vi "Emballage FLATPROP.vi"(2 "error in (no error)":errorcluster caption="entrée d'erreur (pas d'erreur)") -> (0 "error out":errorcluster={"status"=TRUE, "code"=-1, "source"="Fichier des listes de produit vide"} caption="sortie d'erreur")   [LabVIEW 2020]
uses:
  Modules/FS/60_FS_Controles/60_FS_SetGet.ctl
  Labview emballage/enum_ON_OFF_Lecteur.ctl
  41349739-ea89-4dfa-8987-3cac980ec602.vi
  <vilib>/Array/Sort 2D Array - Pop Stack.vi
  <vilib>/Array/Sort 2D Array - Push Stack.vi
  Instance          16 21Saved   Emballage V08 .vi
panel:
  out "Nbr p. dernier carton":i16
  out "NumSem":dbl
  out "Version":string caption="String"
  in  "Certificat":bool
  out "Continuer l'emballage":bool
  out "arreterSerie":bool
  out "pièces EC emballées":string
  out "offset sur code \nbar début index":i32
  out "largeur index":i32
  out "Série en cours?":bool
  out "n° lot à scanner":string
  out "recommencer la cmde EC":bool
  out "#valve déjà emballée":i32
  out "Tableau lots OUT":string[][](array[string])
  out "index commande en cours":i32
  out "Etat":T1(ring)
  out "ID Employe":string
  out "Commande interne":bool
  in  "Imprimer n° cmde":bool
  out "Commande":string
  in  "quitter":bool
  in  "historique":bool
  in  "EC emballage":bool
  in  "carton":bool
  out "Article":string
  out "Nom":string
  out "Nombre de pièce":i16
  out "Numéro carton":i16
  out "Numéro scanné":string
  # "Emballage BDD"
  # "Init"
  # "VerificationSerie"
  # "PieceScannee"
  # "VerificationSerie"
  # "Version"
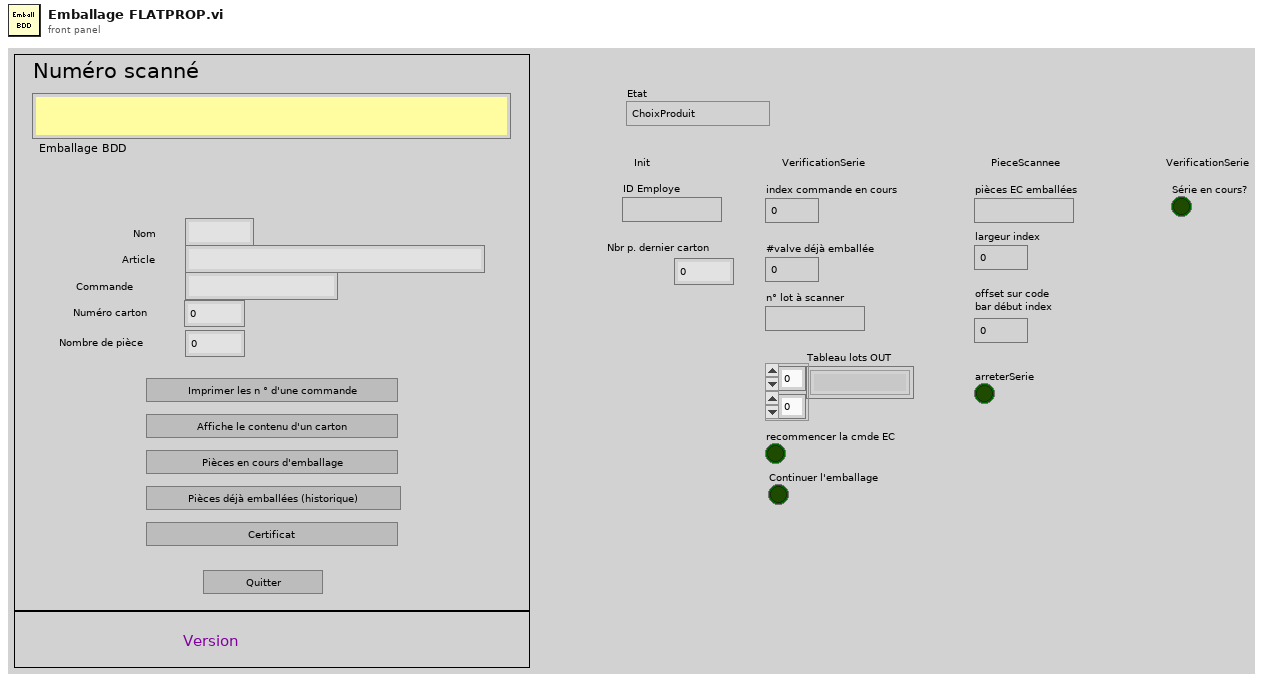
[diagram p1: front panel]
types:
  T1 = enum16{"ChoixProduit", "Init", "VerificationSerie", "LecteurON", "PieceScannee", "LecteurOFF", "SaveData"}
  T2 = typedef "60_FS_SetGet.ctl" = enum16{"set", "get"}
  T3 = typedef "DATA commande.ctl" = cluster{"n°article FAS":string, "n° cmde FAS":string, "quantité cmde":string, "ID LIG cmde":string, "n° cmde client":string, "nom client":string, "n° article client":string, "indice revision client":string, "société de facturation":string, "langue a utiliser":string}
  T4 = typedef "enum_ON_OFF_Lecteur.ctl" = enum16{"ON_COURT", "OFF", "ON", "OFF (open/Close)", "ON (open/close)"}
  T5 = enum16{"n° produit", "date", "opérateur", "n° cmde", "n° carton", "qtté cmdée ou retour client"}
  T6 = enum16{"open", "replace", "create", "open or create", "replace or create", "replace or create with confirmation"}
  T7 = typedef "Emballage_BDD_param_Produit.ctl" = cluster{"No_Valve_FAS":string, "suffixe":string, "designation":string, "indice_produit":string, "code_barre_fixe":string, "affiche_code_barre_client":string, "affiche_no_client":string, "Nb_vlve_par_carton":u16, "melange_des_lots_possible":string, "id_article":string, "Indice_Rev":string, "Famille":string, "date":string, "code_barre_fixe_Fin":string, "Longeur_No_Serie":string}
  T8 = cluster{"ID Employe":string, "NOM ":string, "Code ID Employe":string, "abreviation":string}
  T9 = typedef "60_FS_CLT_Chemins.ctl" = cluster{"Racine_local":path, "Racine_reseau":path, "Racine_Support_Application":path, "Fichier_Journalisation":path, "Connexion_BDD_VSX":path, "Connexion_BDD_PLZ":path}
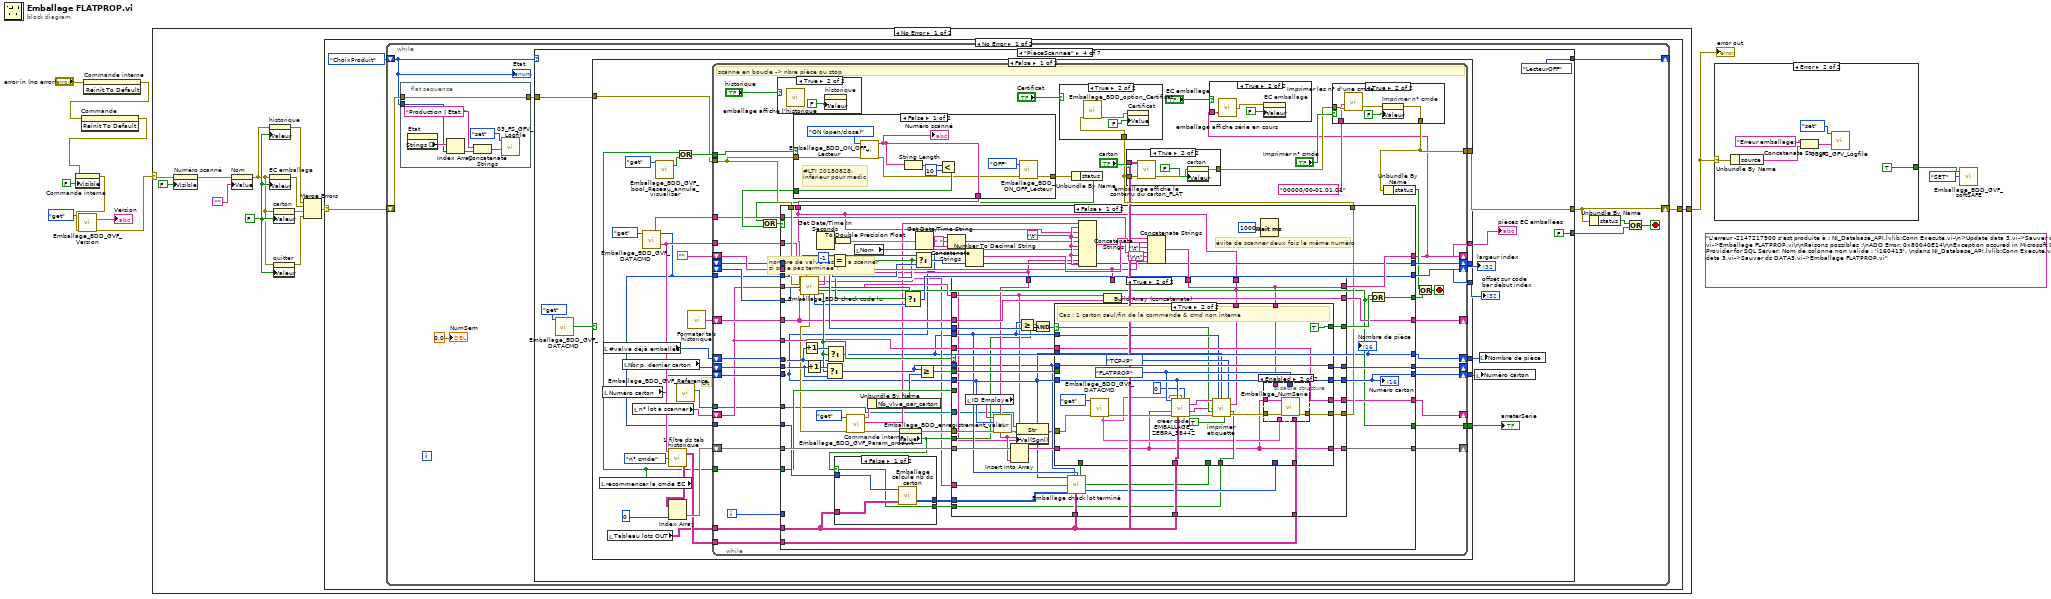
[diagram p0: block diagram]
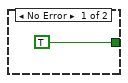
[diagram p2: hidden frame]
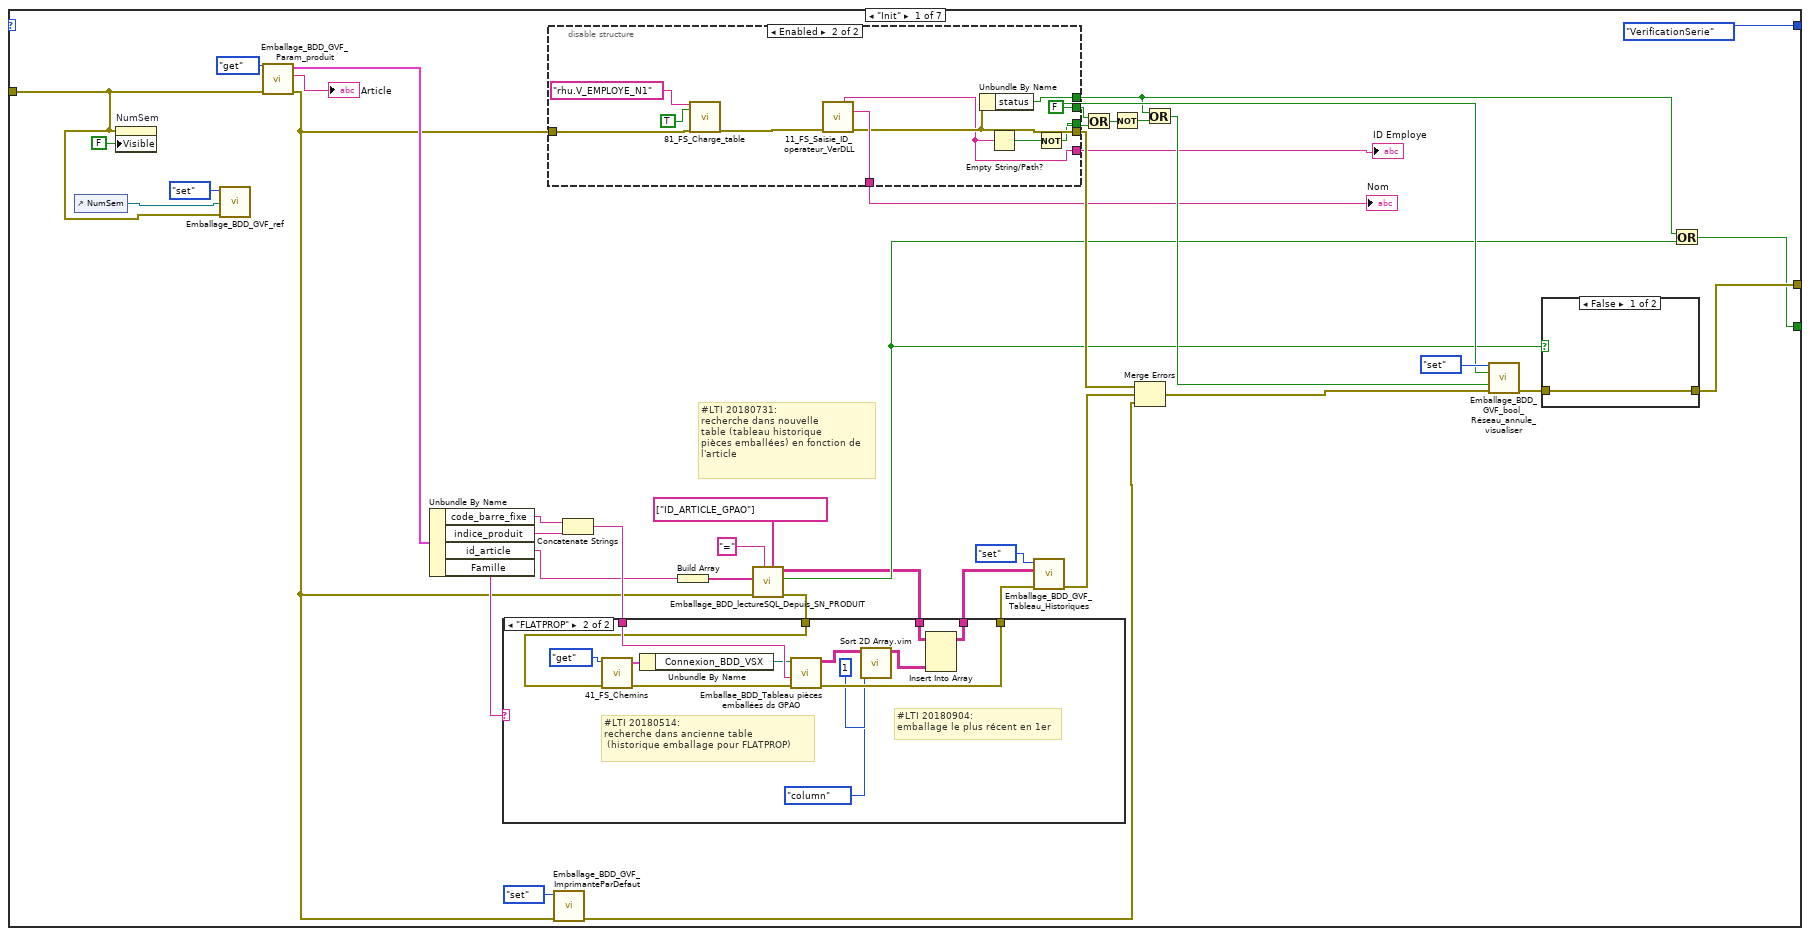
[diagram p3: hidden frame]
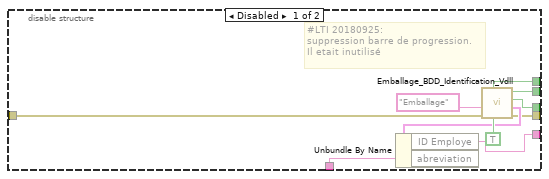
[diagram p4: hidden frame]
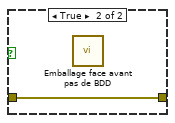
[diagram p6: hidden frame]
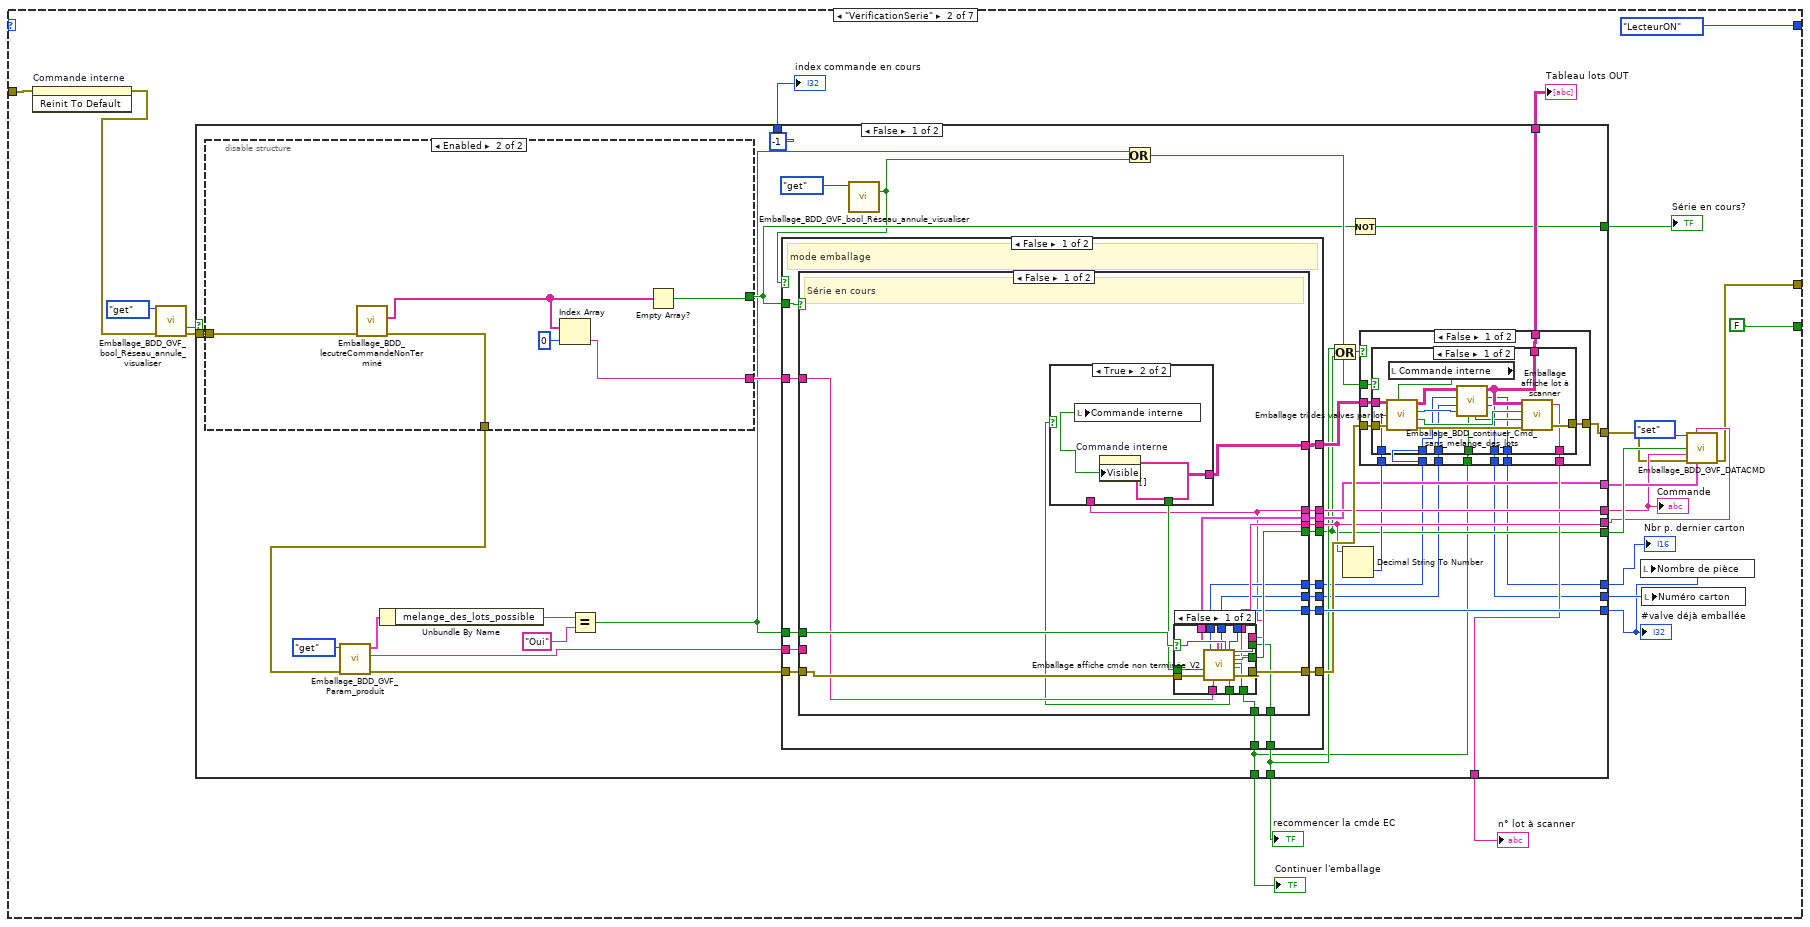
[diagram p7: hidden frame]
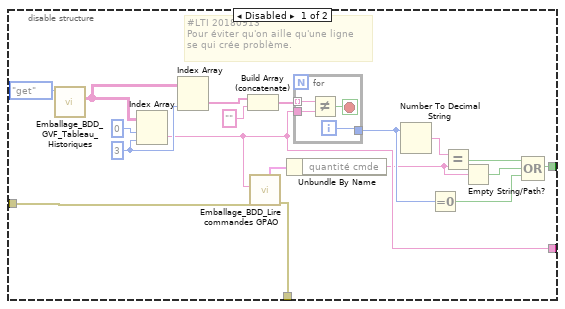
[diagram p8: hidden frame]
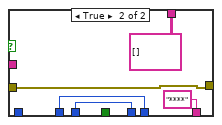
[diagram p9: hidden frame]
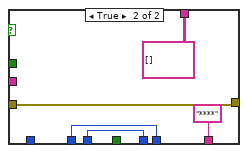
[diagram p10: hidden frame]
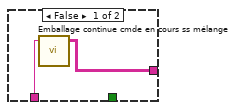
[diagram p11: hidden frame]
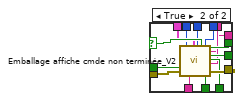
[diagram p12: hidden frame]
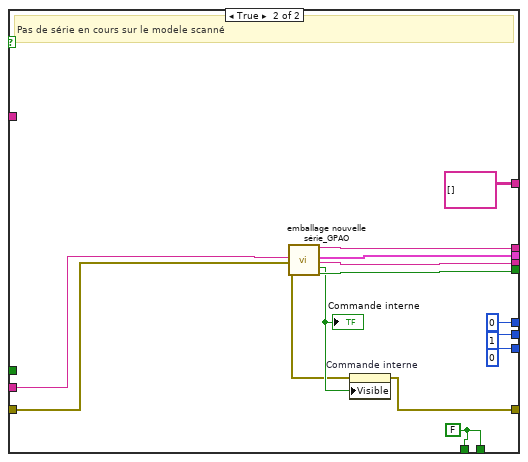
[diagram p13: hidden frame]
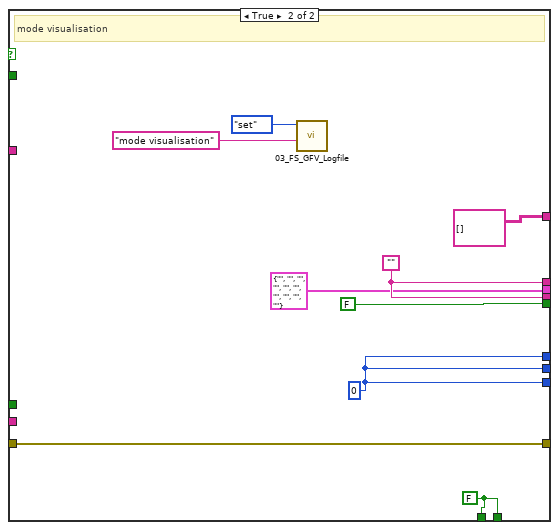
[diagram p14: hidden frame]
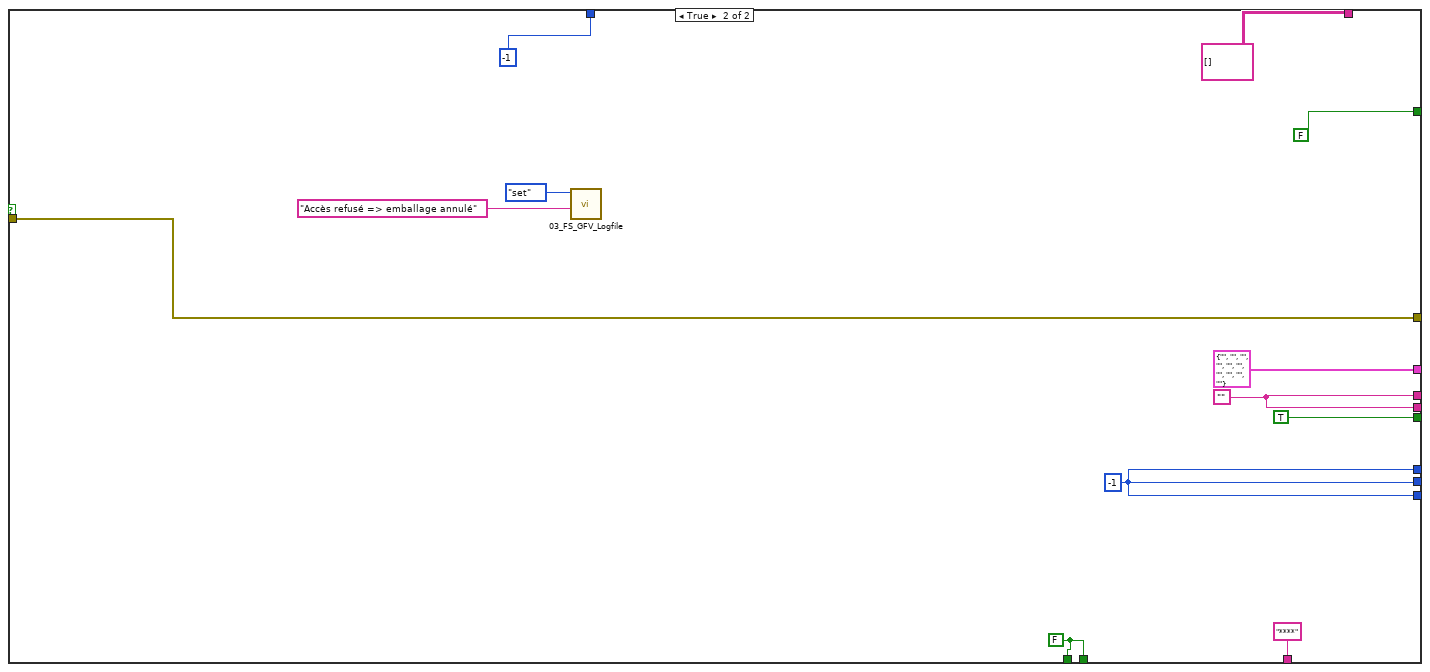
[diagram p15: hidden frame]
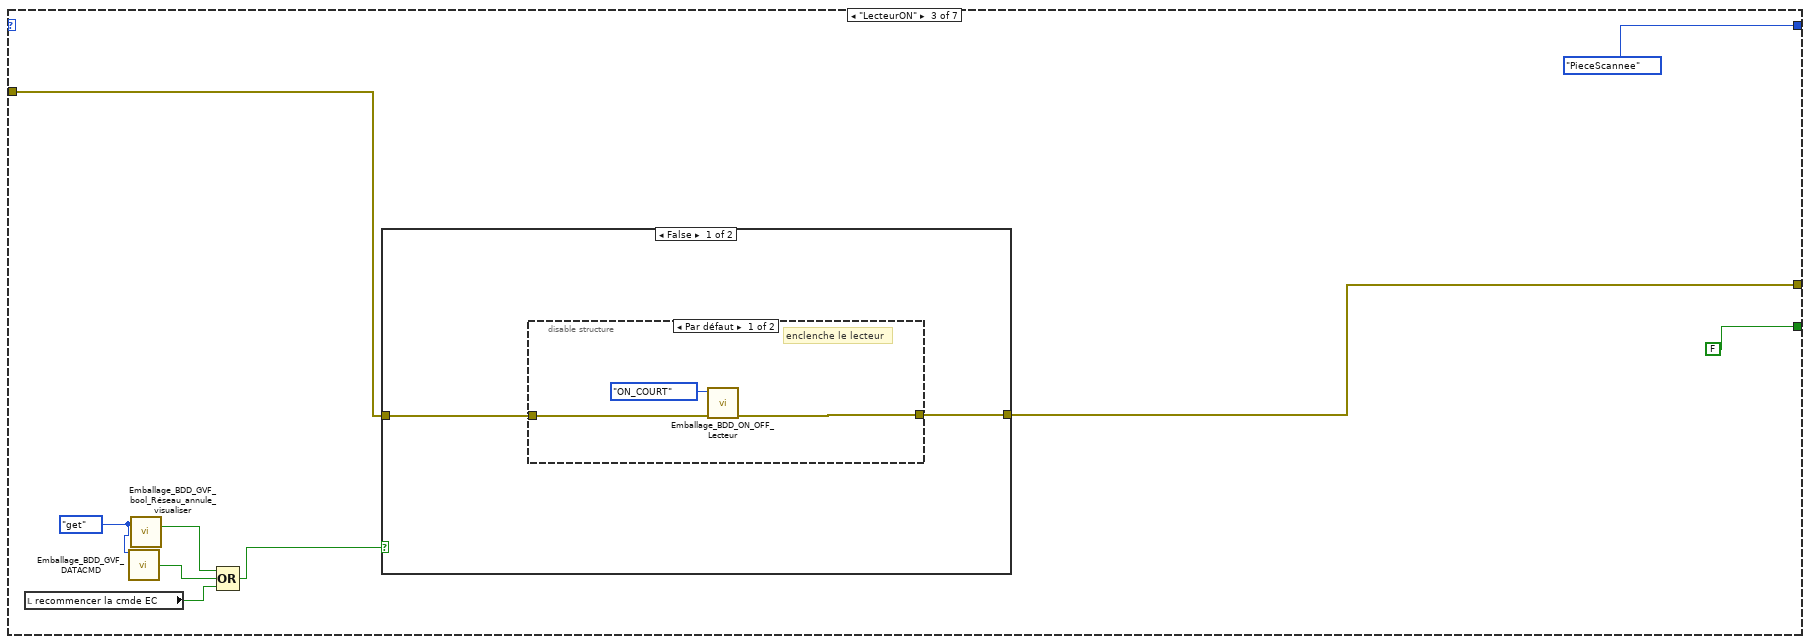
[diagram p16: hidden frame]
diagram:
  (unwired) "L'erreur -2147217900 s'est produite à : NI_Database_API.lvlib:Conn Execute.vi-\n>Update data 3.vi->Sauver ds DATA3.vi->Emballage FLATPROP.vi\r\nRaisons possibles :\nADO Error: 0x80040E14\r\nException occured in Microsoft OLE DB Provider for SQL Server: Nom de colonne non valide : 'i160413'. \ndans NI_Database_API.lvlib:Conn Execute.vi->Update data 3.vi->Sauver ds DATA3.vi->Emballage FLATPROP.vi" ("Explanation")
  n1 = invoke on="Commande interne" class="Bool (strict)" method="Reinit To Default"(error in="error in (no error)") -> (error out=w9:errorcluster)  [unwired: 2 in, 2 out]
  n2 = invoke on="Commande" class="Ch" method="Reinit To Default"(error in=w9) -> (error out=w8:errorcluster)  [unwired: 2 in, 2 out]
  n3 = property on="Commande interne" class="Bool (strict)"(error in=w8, "Visible"=FALSE) -> (error out=w4:errorcluster)  [unwired: 1 in, 1 out]
  n4 = call "Emballage_BDD_GVF_Version.vi"("SetGet"=60_FS_SetGet."get", "Error in"=w4) -> ("Version OUT"=→"Version":string, "Error out"=w3:errorcluster)  [unwired: 12 in]
  n5 = case shown="No Error" w3 {
    selector: w3 -> [w20 w866]
    tunnel: [w23 w866] -> w5
    frame No Error {
      w18 = FALSE
      n6 = property on="Numéro scanné" class="Str"(error in=w20, "Visible"=FALSE) -> (error out=w19:errorcluster)  [unwired: 1 in, 1 out]
      n7 = property on="Nom" class="Str"(error in=w19, "Value"="") -> (error out=w17:errorcluster)  [unwired: 1 in, 1 out]
      n8 = property on="historique" class="Bool (strict)"(error in=w17, "Valeur"=w18) -> (error out=w16:errorcluster)  [unwired: 1 in, 1 out]
      n9 = property on="EC emballage" class="Bool (strict)"(error in=w17, "Valeur"=w18) -> (error out=w15:errorcluster)  [unwired: 1 in, 1 out]
      n10 = property on="carton" class="Bool (strict)"(error in=w17, "Valeur"=w18) -> (error out=w14:errorcluster)  [unwired: 1 in, 1 out]
      n11 = property on="quitter" class="Bool (strict)"(error in=w17, "Valeur"=w18) -> (error out=w13:errorcluster)  [unwired: 1 in, 1 out]
      n12 = Merge Errors(w16, w15, w14, w13) -> (w12:errorcluster)
      n13 = case shown="No Error" w12 {
        selector: w12 -> [w26 w863]
        tunnel: [w25 w863] -> w23
        frame No Error {
          n14 = while {
            shift-right: [w35] -> w25
            shift-left: w26 -> [w30]
            shift-right: [w31] -> _
            shift-left: T1."ChoixProduit" ("Énum") -> [w28]
            stop <- w33 stop-if-true
            n15 = flat-sequence {
              tunnel: w30 -> [w41]
              tunnel: [w41] -> w29
              tunnel: w28 -> [w37]
              frame #0 {
                n16 = property on="Etat" class="Enum (strict)"() -> ("Strings []"=w38:string[])  [unwired: 2 in, 2 out]
                n17 = Index Array(array=w38, index=w37) -> (element=w36:string)
                n18 = Concatenate Strings("Production | Etat: " ("chaîne"), w36) -> (w40:string)
                n19 = call "03_FS_GFV_Logfile.vi"("Chaîne"=w40, "States"=60_FS_SetGet."set") -> ()  [unwired: 8 in, 2 out]
              }
            }
            n20 = case shown="\"PieceScannee\"" w28 {
              tunnel: w29 -> [w48 w124 w350 w372 _ _ w858]
              tunnel: [w64 w125 w349 w364 w726 w774 w857] -> w35
              tunnel: [w63 FALSE ("Erreur de  comunication") FALSE ("Erreur de  comunication") FALSE ("Erreur de  comunication") FALSE ("Erreur de  comunication") w772 w855] -> w32
              tunnel: [T1."VerificationSerie" ("Énum") T1."LecteurON" ("Énum") T1."PieceScannee" ("Énum") T1."LecteurOFF" ("Énum") T1."SaveData" ("Énum") T1."ChoixProduit" ("Énum") T1."Init" ("Énum")] -> w31
              frame "Init" {
                # "#LTI 20180731:\nrecherche dans nouvelle\ntable (tableau historique \npièces emballées) en fonction de\nl'article"
                n21 = control-ref of="NumSem"() -> (w49:refnum<vi>)
                n22 = property on="NumSem" class="DigNum (strict)"(error in=w48, "Visible"=FALSE) -> ()  [unwired: 1 in, 2 out]
                n23 = call "Emballage_BDD_GVF_ref.vi"("Error in"=w48, "Refnum Numsem"=w49, "Énum"=enum16{"set", "get"}."set") -> ()  [unwired: 7 in, 2 out]
                n24 = call "Emballage_BDD_GVF_Param_produit.vi"("Error in"=w48, "Énum"=enum16{"set", "get"}."get") -> ("Error out"=w44:errorcluster, "Produit OUT"=→"Article":string, "CLS_param_produit"=w73:T7)  [unwired: 6 in, 1 out]
                n25 = Unbundle By Name(w73) -> ("code_barre_fixe"=w82:string, "indice_produit"=w81:string, "id_article"=w56:string, "Famille"=w53:string)
                n26 = disable-structure shown="Enabled" {
                  disable-tunnel: [w89 w94] -> w77
                  disable-tunnel: [w88 w98] -> w76
                  disable-tunnel: [w87 FALSE ("Visualiser IN")] -> w68
                  disable-tunnel: [w86 w97] -> w62
                  disable-tunnel: w44 -> [w85 w101]
                  disable-tunnel: [w84 w93] -> w47
                  disable-tunnel: [w83 w99] -> w46
                  frame Disabled {
                    # "#LTI 20180925:\nsuppression barre de progression.\nIl etait inutilisé"
                    n27 = call "Emballage_BDD_Identification_Vdll.vi"("lecture seul possible ?"=TRUE, "error in"=w85, "Posage choisi"="Emballage") -> ("error Out"=w88:errorcluster, "Employe selectionne"=w91:T8, "OK"=w89:bool, "lecture seul"=w87:bool, "Annulé"=w86:bool)  [unwired: 4 in]
                    n28 = Unbundle By Name(w91) -> ("ID Employe"=w84:string, "abreviation"=w83:string)
                  }
                  frame Enabled {
                    n29 = call "81_FS_Charge_table.vi"("table à charger"="rhu.V_EMPLOYE_N1", "T:VSX/F:PLZ"=TRUE, "error in (no error)"=w101) -> ("error out"=w100:errorcluster)  [unwired: 16 in]
                    n30 = call "11_FS_Saisie_ID_operateur_VerDLL.vi"("error in (no error)"=w100) -> ("ID_EMPLOYE"=w93:string, "Visa_employe"=w99:string, "error out"=w98:errorcluster)  [unwired: 9 in, 3 out]
                    n31 = Unbundle By Name(w98) -> ("status"=w97:bool)
                    n32 = Empty String/Path?(string/path=w93) -> (empty?=w95:bool)
                    n33 = Not(x=w95) -> (.not. x?=w94:bool)
                  }
                }
                "Nom" <- w46
                "ID Employe" <- w47
                n34 = call "Emballage_BDD_GVF_ImprimanteParDefaut.vi"("Error in"=w44, "SetGet"=60_FS_SetGet."set") -> ("Error out"=w45:errorcluster)  [unwired: 8 in, 1 out]
                n35 = Concatenate Strings(w82, w81) -> (w80:string)
                n36 = Build Array(w56) -> (w52:string[])
                n37 = call "Emballage_BDD_lectureSQL_Depuis_SN_PRODUIT.vi"("Where (Champs:SN_PRODUIT)"=string[] ["ID_ARTICLE_GPAO"], "Where (Like/=)"="=", "Error in"=w44, "Where (Valeur)"=w52) -> ("Error out"=w58:errorcluster, "Erreur de  comunication"=w60:bool, "Donnees"=w55:string[][])  [unwired: 5 in]
                n38 = case shown="\"FLATPROP\"" w53 {
                  tunnel: w80 -> [_ w118]
                  tunnel: [w105 w113] -> w59
                  tunnel: w58 -> [w105 w112]
                  tunnel: w55 -> [w104 w108]
                  tunnel: [w104 w106] -> w54
                  frame "Faux", Default {
                  }
                  frame "FLATPROP" {
                    # "#LTI 20180904:\nemballage le plus récent en 1er"
                    # "#LTI 20180514:\nrecherche dans ancienne table\n (historique emballage pour FLATPROP)"
                    n39 = call "41_FS_Chemins.vi"("error in (no error)"=w112, "SetGet"=60_FS_SetGet."get") -> ("error out"=w114:errorcluster, "CLT_Chemins_out"=w117:T9)  [unwired: 8 in]
                    n40 = Unbundle By Name(w117) -> ("Connexion_BDD_VSX"=w115:path)
                    n41 = call "Emballae_BDD_Tableau pièces emballées ds GPAO.vi"("error in (no error)"=w114, "Code bar fixe avec indice"=w118, "connection information"=w115) -> ("error out"=w113:errorcluster, "Tableau historique"=w111:string[][])  [unwired: 6 in, 1 out]
                    n42 = call "Sort 2D Array.vim"("index"=1, "dimension to index (column)"=enum16{"column", "row"}."column", "2D array"=w111) -> ("sorted 2D array"=w107:string[][])  [unwired: 7 in, 1 out]
                    n43 = Insert Into Array(array=w108, new element=w107) -> (w106:string[][])  [unwired: 2 in]
                  }
                }
                n44 = call "Emballage_BDD_GVF_Tableau_Historiques.vi"("Error in"=w59, "Tableau historique IN"=w54, "SetGet"=60_FS_SetGet."set") -> ("Error out"=w72:errorcluster)  [unwired: 7 in, 1 out]
                n45 = Or(x=w68, y=w77) -> (x .or. y?=w78:bool)
                n46 = Not(x=w78) -> (.not. x?=w79:bool)
                n47 = Merge Errors(w76, w72, w45) -> (w70:errorcluster)
                n48 = Or(x=w62, y=w79) -> (x .or. y?=w67:bool)
                n49 = call "Emballage_BDD_GVF_bool_Réseau_annule_visualiser.vi"("SetGet"=60_FS_SetGet."set", "Visualiser IN"=w68, "annuler le test car pas d'accès (T) IN"=w67, "Error in"=w70) -> ("Error out"=w65:errorcluster)  [unwired: 9 in, 2 out]
                n50 = case shown="False" w60 {
                  tunnel: [w119 w120] -> w64
                  tunnel: w65 -> [w119 w120]
                  frame False {
                  }
                  frame True {
                    n51 = call "Emballage face avant pas de BDD.vi"() -> ()  [unwired: 4 in, 4 out]
                  }
                }
                n52 = Or(x=w62, y=w60) -> (x .or. y?=w63:bool)
              }
              frame "VerificationSerie" {
                n53 = invoke on="Commande interne" class="Bool (strict)" method="Reinit To Default"(error in=w124) -> (error out=w123:errorcluster)  [unwired: 2 in, 2 out]
                n54 = call "Emballage_BDD_GVF_bool_Réseau_annule_visualiser.vi"("SetGet"=60_FS_SetGet."get", "Error in"=w123) -> ("annuler le test car pas d'accès (T) OUT"=w137:bool, "Error out"=w127:errorcluster)  [unwired: 11 in, 1 out]
                n55 = case shown="False" w137 {
                  tunnel: [w172 w344] -> w133
                  tunnel: [w171 w344] -> w129
                  tunnel: [w164 TRUE] -> w135
                  tunnel: [w148 w343] -> w143
                  tunnel: [w150 w343] -> w122
                  tunnel: [w177 w343] -> w121
                  tunnel: [w175 w342] -> w126
                  tunnel: w127 -> [w153 w342]
                  tunnel: [w157 FALSE] -> w142
                  tunnel: [-1 ("index of element") -1 ("index of element")] -> w141
                  tunnel: [w173 string[][] [] ("Tableau \nlots OUT")] -> w140
                  tunnel: [w169 "****" ("n° lot à scanner")] -> w139
                  tunnel: [w166 w337] -> w128
                  tunnel: [w167 T3 {"n°article FAS"="", "n° cmde FAS"="", "quantité cmde"="", "ID LIG cmde"="", "n° cmde client"="", "nom client"="", "n° article client"="", "indice revision client"="", "société de facturation"="", "langue a utiliser"=""} ("DATA cmde")] -> w134
                  tunnel: [w152 w337] -> w130
                  frame False {
                    n56 = disable-structure shown="Enabled" {
                      disable-tunnel: [w189 w200] -> w156
                      disable-tunnel: [w188 w204] -> w155
                      disable-tunnel: [w185 w203] -> w154
                      disable-tunnel: w153 -> [w180 w205]
                      frame Disabled {
                        w193 = 3 ("indice désactivé (col)")
                        # "#LTI 20180913\nPour éviter qu'on aille qu'une ligne\nse qui crée problème."
                        n57 = call "Emballage_BDD_GVF_Tableau_Historiques.vi"("SetGet"=60_FS_SetGet."get") -> ("Tableau historique OUT"=w179:string[][])  [unwired: 9 in, 1 out]
                        n58 = Index Array(array=w179, index (row)=0 ("indice (ligne)"), index (col)=w193) -> (element=w189:string)
                        n59 = Index Array(array=w179, index (col)=w193) -> (element=w192:string[])  [unwired: 1 in]
                        n60 = Build Array (concatenate)(w192, "" ("DATE_EMBALLAGE")) -> (w183:string[])
                        n61 = call "Emballage_BDD_Lire  commandes GPAO.vi"("error in"=w180, "Numéro commande"=w189) -> ("error out"=w188:errorcluster, "DATA cmde"=w191:T3)  [unwired: 4 in, 4 out]
                        n62 = Unbundle By Name(w191) -> ("quantité cmde"=w184:string)
                        n63 = for {
                          tunnel: w183 -> [w199] mode=indexing
                          tunnel: w189 -> [w198]
                          tunnel: [w196] -> w187
                          i -> [w196]
                          stop <- w197 stop-if-true
                          n64 = Not Equal?(x=w199, y=w198) -> (x != y?=w197:bool)
                        }
                        n65 = Number To Decimal String(number=w187) -> (decimal integer string=w190:string)  [unwired: 1 in]
                        n66 = Equal To 0?(x=w187) -> (x = 0?=w178:bool)
                        n67 = Equal?(x=w190, y=w184) -> (x = y?=w186:bool)
                        n68 = Empty String/Path?(string/path=w184) -> (empty?=w181:bool)
                        n69 = Compound Arithmetic op=OR ("Opérateur arithmétique")(w186, w181, w178) -> (w185:bool)
                      }
                      frame Enabled {
                        n70 = call "Emballage_BDD_lecutreCommandeNonTerminé.vi"("entrée d'erreur (pas d'erreur)"=w205) -> ("sortie d'erreur"=w204:errorcluster, "Cmd_nonFini"=w202:string[])  [unwired: 8 in, 1 out]
                        n71 = Index Array(array=w202, index=0 ("indice")) -> (element=w200:string)
                        n72 = Empty Array?(array=w202) -> (empty?=w203:bool)
                      }
                    }
                    n73 = call "Emballage_BDD_GVF_Param_produit.vi"("Error in"=w155, "Énum"=enum16{"set", "get"}."get") -> ("Error out"=w158:errorcluster, "Produit OUT"=w160:string, "CLS_param_produit"=w159:T7)  [unwired: 6 in, 1 out]
                    n74 = Unbundle By Name(w159) -> ("melange_des_lots_possible"=w163:string)
                    n75 = Equal?(x=w163, y="Oui") -> (x = y?=w144:bool)
                    n76 = call "Emballage_BDD_GVF_bool_Réseau_annule_visualiser.vi"("SetGet"=60_FS_SetGet."get") -> ("Visualiser OUT"=w146:bool)  [unwired: 12 in, 2 out]
                    n77 = case shown="False" w146 {
                      tunnel: w154 -> [w260 _]
                      tunnel: [w259 w329] -> w172
                      tunnel: [w258 w329] -> w171
                      tunnel: [w257 FALSE] -> w164
                      tunnel: [w256 w333] -> w149
                      tunnel: [w255 w333] -> w151
                      tunnel: [w254 w333] -> w177
                      tunnel: w160 -> [w253 _]
                      tunnel: w158 -> [w252 w331]
                      tunnel: [w251 w331] -> w174
                      tunnel: w144 -> [w250 _]
                      tunnel: [w249 string[][] [] ("Tableau des lots déjà emballés")] -> w168
                      tunnel: [w248 w327] -> w166
                      tunnel: [w247 T3 {"n°article FAS"="", "n° cmde FAS"="", "quantité cmde"="", "ID LIG cmde"="", "n° cmde client"="", "nom client"="", "n° article client"="", "indice revision client"="", "société de facturation"="", "langue a utiliser"=""} ("DATA cmde")] -> w167
                      tunnel: [w246 w327] -> w152
                      tunnel: w156 -> [w245 _]
                      frame False {
                        # "mode emballage"
                        n78 = case shown="False" w260 {
                          tunnel: [w261 w324] -> w259
                          tunnel: [w265 w322] -> w258
                          tunnel: [w276 w323] -> w257
                          tunnel: [w262 1] -> w256
                          tunnel: [w264 0] -> w255
                          tunnel: [w263 0] -> w254
                          tunnel: w253 -> [_ w318]
                          tunnel: w252 -> [w275 w314]
                          tunnel: [w274 w317] -> w251
                          tunnel: w250 -> [w273 _]
                          tunnel: [w266 string[][] [] ("Tableau des lots déjà emballés")] -> w249
                          tunnel: [w272 w311] -> w248
                          tunnel: [w271 w315] -> w247
                          tunnel: [w270 w311] -> w246
                          tunnel: w245 -> [w269 _]
                          frame False {
                            # "Série en cours"
                            n79 = case shown="False" w273 {
                              selector: w273 -> [w291 w306]
                              tunnel: w269 -> [w293 w310]
                              tunnel: w275 -> [w295 w309]
                              tunnel: [w294 w308] -> w274
                              tunnel: [w292 w307] -> w272
                              tunnel: [w290 w305] -> w271
                              tunnel: [w289 w304] -> w276
                              tunnel: [w288 w303] -> w270
                              tunnel: [w287 w302] -> w268
                              tunnel: [w286 w301] -> w265
                              tunnel: [w285 w300] -> w261
                              tunnel: [w284 w299] -> w267
                              tunnel: [w282 w298] -> w264
                              tunnel: [w283 w297] -> w263
                              tunnel: [w281 w296] -> w262
                              frame False {
                                n80 = call "Emballage affiche cmde non terminée_V2.vi"("error in (no error)"=w295, "N° cmde en cours"=w293, "melange des lots possibles ?"=w291) -> ("DATA cmde"=w290:T3, "Nombre de carton+1 :"=w281:i16, "pièce(s)"=w282:i16, "#valve déjà emballée"=w283:i32, "Commencer Une autre commande OUT"=w287:bool, "Recommencer la commande OUT"=w292:bool, "No commande FAS"=w285:string, "Pb lecture cmde"=w289:bool, "Continuer l'emballage  OUT"=w288:bool, "Quantité de la commande"=w286:string, "Commande interne"=w284:bool, "error out"=w294:errorcluster)  [unwired: 12 in, 1 out]
                              }
                              frame True {
                                n81 = call "Emballage affiche cmde non terminée_V2.vi"("error in (no error)"=w309, "N° cmde en cours"=w310, "melange des lots possibles ?"=w306) -> ("DATA cmde"=w305:T3, "Nombre de carton+1 :"=w296:i16, "pièce(s)"=w298:i16, "#valve déjà emballée"=w297:i32, "Commencer Une autre commande OUT"=w302:bool, "Recommencer la commande OUT"=w307:bool, "No commande FAS"=w300:string, "Pb lecture cmde"=w304:bool, "Continuer l'emballage  OUT"=w303:bool, "Quantité de la commande"=w301:string, "Commande interne"=w299:bool, "error out"=w308:errorcluster)  [unwired: 12 in, 1 out]
                              }
                            }
                            n82 = case shown="True" w268 {
                              tunnel: [w277 string[][] [] ("Tableau des lots déjà emballés")] -> w266
                              tunnel: w267 -> [_ w279]
                              tunnel: w261 -> [w278 _]
                              frame False {
                                n83 = call "Emballage continue cmde en cours ss mélange.vi"("n° cmde"=w278) -> ("Tableau des lots déjà emballés"=w277:string[][])  [unwired: 2 in, 2 out]
                              }
                              frame True {
                                n84 = local write "Commande interne"(w279) -> ()
                                n85 = property on="Commande interne" class="Bool (strict)"("Visible"=w279) -> ()  [unwired: 2 in, 2 out]
                              }
                            }
                          }
                          frame True {
                            w311 = FALSE ("Terminer la commande OUT")
                            # "Pas de série en cours sur le modele scanné"
                            n86 = call "emballage nouvelle série_GPAO.vi"("Nom du produit"=w318, "error in (no error)"=w314) -> ("error out"=w312:errorcluster, "No commande FAS"=w324:string, "DATA cmde"=w315:T3, "Quantité de la commande"=w322:string, "Commande interne"=w313:bool, "Annuler(T=OK)"=w323:bool)  [unwired: 11 in, 1 out]
                            "Commande interne" <- w313
                            n87 = property on="Commande interne" class="Bool (strict)"(error in=w312, "Visible"=w313) -> (error out=w317:errorcluster)  [unwired: 1 in, 1 out]
                          }
                        }
                      }
                      frame True {
                        w327 = FALSE ("Terminer la commande OUT")
                        w329 = ""
                        w333 = 0
                        # "mode visualisation"
                        n88 = call "03_FS_GFV_Logfile.vi"("Chaîne"="mode visualisation", "States"=60_FS_SetGet."set") -> ()  [unwired: 8 in, 2 out]
                      }
                    }
                    n89 = Or(x=w144, y=w146) -> (x .or. y?=w162:bool)
                    n90 = Or(x=w166, y=w164) -> (x .or. y?=w165:bool)
                    n91 = Decimal String To Number(string=w171) -> (number=w170:i32)  [unwired: 2 in, 1 out]
                    n92 = Not(x=w154) -> (.not. x?=w157:bool)
                    n93 = case shown="False" w165 {
                      tunnel: [w217 w244] -> w175
                      tunnel: w174 -> [w216 w244]
                      tunnel: [w215 string[][] [] ("Tableau \nlots OUT")] -> w173
                      tunnel: w162 -> [w214 _]
                      tunnel: w170 -> [w213 _]
                      tunnel: [w212 "****" ("n° lot à scanner")] -> w169
                      tunnel: w168 -> [w211 _]
                      tunnel: w149 -> [w210 w241]
                      tunnel: w151 -> [w209 w240]
                      tunnel: w152 -> [w208 _]
                      tunnel: [w207 w240] -> w150
                      tunnel: [w206 w241] -> w148
                      frame False {
                        n94 = case shown="False" w214 {
                          tunnel: w216 -> [w232 w239]
                          tunnel: [w234 w239] -> w217
                          tunnel: [w227 string[][] [] ("Tableau \nlots OUT")] -> w215
                          tunnel: w213 -> [w231 _]
                          tunnel: [w230 "****" ("n° lot à scanner")] -> w212
                          tunnel: w211 -> [w229 _]
                          tunnel: w210 -> [w223 w236]
                          tunnel: w209 -> [w222 w235]
                          tunnel: w208 -> [w221 _]
                          tunnel: [w220 w235] -> w207
                          tunnel: [w219 w236] -> w206
                          frame False {
                            n95 = local read "Commande interne"() -> (w218:bool)
                            n96 = call "Emballage tri des valves par lot.vi"("Tableau lots IN"=w229, "Commande interne"=w218, "TOTAL à atteindre :"=w231, "error in (no error)"=w232) -> ("Tableau lots OUT"=w226:string[][], "indice n° lot a scanner"=w225:u64, "Bouton confimer OUT"=w228:bool, "error out"=w233:errorcluster)  [unwired: 3 in]
                            n97 = call "Emballage_BDD_continuer_Cmd_sans_melange_des_lots.vi"("Continuer?"=w221, "indice lot IN"=w225, "Numero carton IN"=w223, "Nombre de pièce \nds dernier carton IN"=w222, "Tableau lots OUT"=w226) -> ("indice lot OUT"=w224:i32, "Numero carton OUT"=w219:i32, "Nombre de pièce ds dernier carton OUT"=w220:i32, "Tableau lots OUT 2"=w227:string[][])  [unwired: 3 in]
                            n98 = call "Emballage affiche lot à scanner.vi"("Tableau \nlots OUT"=w227, "Affiche ?"=w228, "Indice n° lot à scanner"=w224, "error in (no error)"=w233) -> ("n° lot à scanner"=w230:string, "error out"=w234:errorcluster)  [unwired: 1 in, 1 out]
                          }
                          frame True {
                          }
                        }
                      }
                      frame True {
                      }
                    }
                  }
                  frame True {
                    w337 = FALSE ("Terminer la commande OUT")
                    w343 = -1
                    w344 = ""
                    n99 = call "03_FS_GFV_Logfile.vi"("Chaîne"="Accès refusé => emballage annulé", "States"=60_FS_SetGet."set") -> ()  [unwired: 8 in, 2 out]
                  }
                }
                "Commande" <- w133
                "index commande en cours" <- w141
                "Tableau lots OUT" <- w140
                "#valve déjà emballée" <- w121
                "recommencer la cmde EC" <- w128
                "n° lot à scanner" <- w139
                "Série en cours?" <- w142
                "Continuer l'emballage" <- w130
                "Nbr p. dernier carton" <- w122
                n100 = local write "Nombre de pièce"(w121) -> ()
                n101 = local write "Numéro carton"(w143) -> ()
                n102 = call "Emballage_BDD_GVF_DATACMD.vi"("SetGet"=60_FS_SetGet."set", "Quantité de la commande IN"=w129, "Annuler new série (T=OK) IN"=w135, "No commande FAS IN"=w133, "Error in"=w126, "DATA cmde IN"=w134) -> ("Error out"=w125:errorcluster)  [unwired: 2 in, 7 out]
              }
              frame "LecteurON" {
                w351 = 60_FS_SetGet."get" ("SetGet")
                n103 = local read "recommencer la cmde EC"() -> (w348:bool)
                n104 = call "Emballage_BDD_GVF_DATACMD.vi"("SetGet"=w351) -> ("Annuler new série (T=OK) OUT"=w352:bool)  [unwired: 7 in, 7 out]
                n105 = call "Emballage_BDD_GVF_bool_Réseau_annule_visualiser.vi"("SetGet"=w351) -> ("Visualiser OUT"=w353:bool)  [unwired: 12 in, 2 out]
                n106 = Compound Arithmetic op=OR(w353, w352, w348) -> (w354:bool)
                n107 = case shown="False" w354 {
                  tunnel: [w356 w361] -> w349
                  tunnel: w350 -> [w355 w361]
                  frame False {
                    n108 = disable-structure shown="Par défaut" {
                      disable-tunnel: [w358 w360] -> w356
                      disable-tunnel: w355 -> [w359 w360]
                      frame condition #0 (active) {
                        # "enclenche le lecteur"
                        n109 = call "Emballage_BDD_ON_OFF_Lecteur.vi"("Error in"=w359, "ON/OFF lecteur"=enum_ON_OFF_Lecteur."ON_COURT") -> ("Error out"=w358:errorcluster)  [unwired: 7 in, 2 out]
                      }
                      frame condition #1 {
                      }
                    }
                  }
                  frame True {
                    # "(pas de scan carte OP)"
                    # "scanner pas lancé"
                  }
                }
              }
              frame "PieceScannee" {
                # "nombre de valve restant a scanner\nsi série pas terminée ?"
                n110 = call "Emballage_BDD_GVF_DATACMD.vi"("SetGet"=60_FS_SetGet."get") -> ("Annuler new série (T=OK) OUT"=w368:bool)  [unwired: 7 in, 7 out]
                n111 = case shown="False" w368 {
                  tunnel: [w402 ""] -> w373
                  tunnel: [w401 w723] -> w364
                  tunnel: w372 -> [w377 w723]
                  tunnel: [w400 w722] -> w366
                  tunnel: [w399 w722] -> w365
                  tunnel: [w382 w722] -> w370
                  tunnel: [w383 w722] -> w371
                  tunnel: [w397 FALSE ("quitter")] -> w367
                  frame False {
                    # "crt"
                    n112 = local read "recommencer la cmde EC"() -> (w380:bool)
                    n113 = local read "Numéro carton"() -> (w379:i16)
                    n114 = local read "#valve déjà emballée"() -> (w378:i32)
                    n115 = local read "Tableau lots OUT"() -> (w381:string[][])
                    n116 = local read "Nbr p. dernier carton"() -> (w374:i16)
                    n117 = local read "n° lot à scanner"() -> (w376:string)
                    n118 = call "Emballage_BDD_GVF_DATACMD.vi"("SetGet"=60_FS_SetGet."get") -> (3:"Quantité de la commande OUT"=w384:string, 4:"Quantité de la commande OUT"=w385:i32, "No commande FAS OUT"=w386:string)  [unwired: 7 in, 5 out]
                    n119 = call "Emballage_BDD_GVF_bool_Réseau_annule_visualiser.vi"("SetGet"=60_FS_SetGet."get") -> ("Visualiser OUT"=w388:bool)  [unwired: 12 in, 2 out]
                    n120 = call "1 filtre ds tab historique.vi"("Filtre"=T5."n° cmde", "valeur recherchée"=w386) -> ("Tab historique filtré par ordre croissant carton"=w390:string[][], "Tab historique filtré"=w394:string[][])  [unwired: 1 in]
                    n121 = Index Array(array=w390, index (col)=0) -> (element=w395:string[])  [unwired: 1 in]
                    n122 = Or(x=w380, y=w388) -> (x .or. y?=w391:bool)
                    n123 = call "Emballage_BDD_GVF_Reference.vi"() -> ("ref piece OUT"=w375:refnum<vi>)  [unwired: 14 in, 1 out]
                    n124 = call "Formater tab historique.vi"() -> ("tab histo reformaté"=w392:string[])  [unwired: 1 in]
                    n125 = while {
                      shift-right: [w410] -> w402
                      shift-left: "" -> [w449]
                      shift-right: [w444] -> w399
                      shift-left: w379 -> [w448]
                      shift-right: [w445] -> _
                      shift-left: w374 -> [w447]
                      tunnel: w385 -> [w412]
                      shift-right: [w441] -> w400
                      shift-left: w378 -> [w446]
                      tunnel: [w416] -> w401
                      shift-right: [w442] -> _
                      shift-left: w392 -> [w443]
                      tunnel: w391 -> [w433]
                      shift-right: [w437] -> w383
                      shift-left: _ -> [w435]
                      shift-right: [w436] -> w382
                      shift-left: _ -> [w434]
                      tunnel: w385 -> [w432]
                      shift-right: [w430] -> _
                      shift-left: w395 -> [w431]
                      tunnel: [w429] -> w397
                      tunnel: w381 -> [w403]
                      tunnel: w380 -> [w427]
                      shift-right: [w426] -> _
                      shift-left: w376 -> [w425]
                      tunnel: w394 -> [w424]
                      tunnel: w386 -> [w423]
                      tunnel: w377 -> [w418]
                      tunnel: w384 -> [w411]
                      tunnel: w375 -> [w404]
                      i -> [w421]
                      stop <- w405 stop-if-true
                      # "scanne en boucle -> nbre pièce ou stop"
                      n126 = case shown="True" "historique" {
                        frame False {
                        }
                        frame True {
                          n127 = call "emballage affiche l'historique.vi"() -> ()  [unwired: 3 in]
                          n128 = property on="historique" class="Bool (strict)"("Valeur"=FALSE) -> ()  [unwired: 2 in, 2 out]
                        }
                      }
                      n129 = case shown="False" w433 {
                        tunnel: [w465 TRUE] -> w413
                        tunnel: [w460 w469] -> w407
                        tunnel: [w462 ""] -> w428
                        tunnel: w418 -> [w463 _]
                        frame False {
                          # "#LTI 20180828:\ninférieur pour medic"
                          n130 = call "Emballage_BDD_ON_OFF_Lecteur.vi"("Error in"=w463, "ON/OFF lecteur"=enum_ON_OFF_Lecteur."ON (open/close)") -> ("Error out"=w461:errorcluster, "Etiquette scanné"=w462:string)  [unwired: 7 in, 1 out]
                          "Numéro scanné" <- w462
                          n131 = String Length(string=w462) -> (length=w466:i32)
                          n132 = Less?(x=w466, y=10) -> (x < y?=w465:bool)
                          n133 = call "Emballage_BDD_ON_OFF_Lecteur.vi"("Error in"=w461, "ON/OFF lecteur"=enum_ON_OFF_Lecteur."OFF") -> ("Error out"=w460:errorcluster)  [unwired: 7 in, 2 out]
                        }
                        frame True {
                          # "en mode uniquement affiche information"
                          n134 = property on="Numéro scanné" class="Str"("Visible"=FALSE) -> (error out=w469:errorcluster)  [unwired: 2 in, 1 out]
                        }
                      }
                      n135 = Unbundle By Name(w407) -> ("status"=w409:bool)
                      n136 = Or(x=w409, y=w413) -> (x .or. y?=w414:bool)
                      n137 = case shown="False" w414 {
                        tunnel: w447 -> [w546 w714]
                        tunnel: [w526 w713] -> w410
                        tunnel: [w538 w704] -> w444
                        tunnel: [w545 w714] -> w445
                        tunnel: w449 -> [w525 w713]
                        tunnel: [w542 w701] -> w417
                        tunnel: w446 -> [w529 w697]
                        tunnel: [w482 w697] -> w441
                        tunnel: w448 -> [w486 w704]
                        tunnel: w428 -> [w487 _]
                        tunnel: [w515 w698] -> w406
                        tunnel: w418 -> [w501 w712]
                        tunnel: w443 -> [w516 w709]
                        tunnel: [w528 w709] -> w442
                        tunnel: w412 -> [w534 _]
                        tunnel: [w521 w708] -> w437
                        tunnel: [w519 w707] -> w436
                        tunnel: w435 -> [w522 w708]
                        tunnel: w434 -> [w518 w707]
                        tunnel: w432 -> [w509 _]
                        tunnel: w431 -> [w513 w705]
                        tunnel: [w514 w705] -> w430
                        tunnel: [w500 "quitter"] -> w429
                        tunnel: w403 -> [w510 _]
                        tunnel: w425 -> [w506 w706]
                        tunnel: w427 -> [w505 w703]
                        tunnel: [w504 w706] -> w426
                        tunnel: w425 -> [w503 _]
                        tunnel: w424 -> [w491 _]
                        tunnel: w423 -> [w489 _]
                        tunnel: w421 -> [_ _]
                        tunnel: w411 -> [w488 _]
                        tunnel: w404 -> [w484 _]
                        frame False {
                          w536 = "\t"
                          # "évite de scanner deux fois le même numéro"
                          n138 = call "Emballage_BDD check code lu.vi"("error in"=w501, "n° lot à scanner"=w506, "chaîne lue par le lecteur IN"=w487, "tab pcs déjà emballées (histo+actu)"=w516, "Quantité du lot de livraison"=w534, "n° commande EC"=w489) -> ("error out"=w493:errorcluster, "offset sur code bar début index"=w520:i16, "largeur index"=w523:i16, "Date production de la piéce"=w483:string, "chaîne lue par le lecteur OUT"=w502:string, "Arrêter la série (T)"=w500:bool, "Paramètres OK(=> T)"=w537:bool)  [unwired: 7 in]
                          n139 = Increment(x=w529) -> (x+1=w541:i32)
                          n140 = Increment(x=w546) -> (x+1=w540:i32)
                          n141 = Get Date/Time In Seconds() -> (seconds since 1Jan1904=w549:timestamp)
                          n142 = Select(t=w540, s=w537, f=w546) -> (s? t:f=w511:i32)
                          n143 = Select(t=w541, s=w537, f=w529) -> (s? t:f=w482:i32)
                          "Nombre de pièce" <- w482
                          n144 = Equal?(x=-1, y=w523) -> (x = y?=w517:bool)
                          n145 = To Double Precision Float(number=w549) -> (double precision float=w548:dbl)
                          n146 = call "Emballage_BDD_GVF_Param_produit.vi"("Error in"=w493, "Énum"=enum16{"set", "get"}."get") -> ("Error out"=w492:errorcluster, "Produit OUT"=w494:string, "CLS_param_produit"=w497:T7)  [unwired: 6 in, 1 out]
                          n147 = local read "Nom"() -> (w495:string)
                          n148 = Unbundle By Name(w497) -> ("Nb_vlve_par_carton"=w496:u16)
                          n149 = property on="Commande interne" class="Bool (strict)"(error in=w492) -> (error out=w499:errorcluster, "Value"=w485:bool)  [unwired: 1 in, 1 out]
                          n150 = case shown="False" w485 {
                            selector: w485 -> [w550 w554]
                            tunnel: w510 -> [w553 _]
                            tunnel: w509 -> [w552 w556]
                            tunnel: [w551 w555] -> w508
                            tunnel: [w550 w554] -> w498
                            frame False {
                              n151 = call "Emballage calcule nb ds carton.vi"("Tableau \nlots OUT"=w553, "Quantité de la cmde"=w552) -> ("Tab n° carton - nb ds carton"=w551:i32[][])  [unwired: 1 in, 1 out]
                            }
                            frame True {
                              n152 = Build Array(1 ("Nbr Carton"), w556) -> (w558:i32[])
                              n153 = Build Array(w558) -> (w555:i32[][])
                            }
                          }
                          n154 = Select(t=w518, s=w517, f=w520) -> (s? t:f=w519:i16)
                          n155 = Select(t=w522, s=w517, f=w523) -> (s? t:f=w521:i16)
                          n156 = Get Date/Time String(seconds (now)=w548) -> (date string=w547:string, time string=w544:string)  [unwired: 2 in]
                          n157 = Greater Or Equal?(x=w511, y=w496) -> (x >= y?=w507:bool)
                          n158 = Concatenate Strings(w547, " ", w544) -> (w512:string)
                          n159 = Number To Decimal String(number=w486) -> (decimal integer string=w531:string)  [unwired: 1 in]
                          n160 = Concatenate Strings(w494, w536, w487, w536, w512, w536, w495, w536, w489, w536) -> (w532:string)
                          n161 = Concatenate Strings(w532, w531, "\t", w488, "\r\n", w525) -> (w527:string)
                          n162 = case shown="True" w537 {
                            tunnel: [w565 w597] -> w538
                            tunnel: w511 -> [w566 w574]
                            tunnel: [w566 w598] -> w545
                            tunnel: w507 -> [_ w599]
                            tunnel: w486 -> [w565 w577]
                            tunnel: w482 -> [_ w581]
                            tunnel: [FALSE w603] -> w530
                            tunnel: w534 -> [_ w602]
                            tunnel: w516 -> [w563 w601]
                            tunnel: [w563 w600] -> w528
                            tunnel: w527 -> [_ w585]
                            tunnel: [w562 w585] -> w526
                            tunnel: w525 -> [w562 _]
                            tunnel: w502 -> [_ w575]
                            tunnel: w513 -> [w560 w594]
                            tunnel: [w561 w596] -> w515
                            tunnel: w499 -> [w561 w579]
                            tunnel: [w560 w595] -> w514
                            tunnel: w489 -> [_ w576]
                            tunnel: w510 -> [_ w593]
                            tunnel: w510 -> [_ w592]
                            tunnel: w508 -> [_ w588]
                            tunnel: w483 -> [_ w586]
                            tunnel: w505 -> [_ _]
                            tunnel: [w559 w584] -> w504
                            tunnel: w503 -> [w559 w583]
                            tunnel: w491 -> [_ w582]
                            tunnel: w498 -> [_ w580]
                            tunnel: w487 -> [_ w568]
                            tunnel: w485 -> [_ w571]
                            tunnel: w484 -> [_ w567]
                            frame False {
                            }
                            frame True {
                              n163 = local read "ID Employe"() -> (w578:string)
                              n164 = call "Emballage_BDD_enregistrement_valeur.vi"("SN_PRODUIT"=w575, "NO_CDEVAL"=w576, "Error in"=w579, "NO_DU_CARTON"=w577, "ID_UTILISATEUR_GPAO"=w578) -> ("Error out"=w570:errorcluster)  [unwired: 6 in]
                              n165 = Insert Into Array(array=w594, new element=w575) -> (w589:string[])  [unwired: 1 in]
                              n166 = property on="Nœud de propriété" class="Str"(reference=w567, error in=w570, "Val(Sgnl)"=w568) -> (error out=w569:errorcluster)  [unwired: 1 out]
                              n167 = Greater Or Equal?(x=w581, y=w602) -> (x >= y?=w572:bool)
                              n168 = Compound Arithmetic op=AND ("Opérateur arithmétique")(w572, invert w571) -> (w573:bool)
                              n169 = call "Emballage check lot terminé.vi"("N° carton en cours"=w577, "Nb valves dans carton"=w574, "Nombre de pièce emballées"=w581, "date de prod de la piece en cours"=w586, "Tab n° carton - nb ds carton"=w588, "Tableau lots OUT"=w592) -> ("Changer de carton"=w587:bool, "Affiche \"scan lot suivant\""=w591:bool, "indice lot suivant"=w590:i32)  [unwired: 7 in]
                              n170 = case shown="True" w573 {
                                selector: w573 -> [w605 w671]
                                tunnel: [FALSE TRUE] -> w603
                                tunnel: w577 -> [_ w675]
                                tunnel: w581 -> [_ w674]
                                tunnel: w599 -> [w611 _]
                                tunnel: w574 -> [w622 w686]
                                tunnel: w577 -> [w621 w683]
                                tunnel: [w620 w686] -> w598
                                tunnel: [w619 w683] -> w597
                                tunnel: w589 -> [w618 w663]
                                tunnel: [w617 w680] -> w596
                                tunnel: w569 -> [w616 w669]
                                tunnel: [w615 w663] -> w595
                                tunnel: w593 -> [w614 w682]
                                tunnel: w591 -> [w613 _]
                                tunnel: w590 -> [w612 _]
                                tunnel: w587 -> [w609 _]
                                tunnel: w585 -> [_ w670]
                                tunnel: [w608 w679] -> w584
                                tunnel: w583 -> [w607 w679]
                                tunnel: w582 -> [_ w678]
                                tunnel: w580 -> [w606 w672]
                                tunnel: w568 -> [w604 w664]
                                frame False {
                                # "cmd non termine ou cmd interne"
                                n171 = Or(x=w611, y=w609) -> (x .or. y?=w610:bool)
                                n172 = case shown="True" w610 {
                                tunnel: w621 -> [w628 w652]
                                tunnel: [w628 w643] -> w619
                                tunnel: w622 -> [w627 _]
                                tunnel: [w627 0] -> w620
                                tunnel: w618 -> [w625 w648]
                                tunnel: [w626 w650] -> w617
                                tunnel: w616 -> [w626 w640]
                                tunnel: [w625 w648] -> w615
                                tunnel: w614 -> [_ w649]
                                tunnel: w613 -> [_ w647]
                                tunnel: w612 -> [_ w646]
                                tunnel: [w624 w645] -> w608
                                tunnel: w607 -> [w624 w644]
                                tunnel: w606 -> [_ w642]
                                tunnel: w605 -> [_ w641]
                                tunnel: w604 -> [_ w636]
                                frame False {
                                }
                                frame True {
                                # "Carton terminé"
                                n173 = call "Emballage_BDD_GVF_DATACMD.vi"("SetGet"=60_FS_SetGet."get", "Error in"=w640) -> ("DATA cmde OUT"=w637:T3, "Error out"=w639:errorcluster)  [unwired: 6 in, 6 out]
                                n174 = Increment(x=w652) -> (x+1=w643:i16)
                                n175 = call "créer code EMBALLAGE_ZEBRA_3844Z.vi"("DIVISION"=enum16{"FLATPROP", "MEDIC"}."FLATPROP", "N° carton"=w652, "DATA cmde"=w637, "Nb total cartons"=0, "Tableau n° valves"=w648, "error in (no error)"=w639, "Tableau \nlots OUT"=w649) -> ("chaine  à écrire"=w634:string, "n°article FAS"=w629:string, "error out"=w635:errorcluster)  [unwired: 5 in, 1 out]
                                n176 = call "imprimer etiquette.vi"("chaine à écrire"=w634, "Type de liaison"=enum16{"RS232", "USB", "TCP-IP", "Aucune"}."TCP-IP", "Bloc Scanné"=w636, "n°article FAS"=w629, "sélecteur"=w641, "Cde_Interne"=w642, "error in"=w635, "Carton Numéro"=w643, "fin de série ?"=FALSE) -> ("error out"=w651:errorcluster)  [unwired: 6 in]
                                n177 = case shown="True" w647 {
                                selector: w647 -> [_ w657]
                                tunnel: w651 -> [w655 w661]
                                tunnel: [w655 w660] -> w650
                                tunnel: w649 -> [_ w659]
                                tunnel: w646 -> [_ w658]
                                tunnel: [w654 w656] -> w645
                                tunnel: w644 -> [w654 _]
                                frame False {
                                }
                                frame True {
                                n178 = call "Emballage affiche lot à scanner.vi"("Tableau \nlots OUT"=w659, "Affiche ?"=w657, "Indice n° lot à scanner"=w658, "error in (no error)"=w661) -> ("n° lot à scanner"=w656:string, "error out"=w660:errorcluster)  [unwired: 1 in, 1 out]
                                }
                                }
                                }
                                }
                                }
                                frame True {
                                w677 = enum16{"FLATPROP", "MEDIC"}."FLATPROP" ("DIVISION")
                                # "Cas : 1 carton seul/fin de la commande & cmd non interne"
                                n179 = call "Emballage_BDD_GVF_DATACMD.vi"("SetGet"=60_FS_SetGet."get", "Error in"=w669) -> ("DATA cmde OUT"=w667:T3, "Error out"=w668:errorcluster)  [unwired: 6 in, 6 out]
                                n180 = call "créer code EMBALLAGE_ZEBRA_3844Z.vi"("DIVISION"=w677, "N° carton"=w683, "DATA cmde"=w667, "Nb total cartons"=0, "Tableau n° valves"=w663, "error in (no error)"=w668, "Tableau \nlots OUT"=w682) -> ("chaine  à écrire"=w684:string, "n°article FAS"=w665:string, "error out"=w685:errorcluster)  [unwired: 5 in, 1 out]
                                n181 = call "imprimer etiquette.vi"("chaine à écrire"=w684, "nbr de valve"=w674, "nbr de carton"=w675, "Type de liaison"=enum16{"RS232", "USB", "TCP-IP"}."TCP-IP", "Bloc Scanné"=w664, "n°article FAS"=w665, "sélecteur"=w671, "Cde_Interne"=w672, "error in"=w685, "fin de série ?"=TRUE) -> ("error out"=w681:errorcluster)  [unwired: 5 in]
                                n182 = disable-structure shown="Enabled" {
                                disable-tunnel: w681 -> [w693 w696]
                                disable-tunnel: [w692 w695] -> w680
                                disable-tunnel: w678 -> [w691 _]
                                disable-tunnel: w677 -> [w690 _]
                                disable-tunnel: w670 -> [w689 _]
                                disable-tunnel: w667 -> [w688 _]
                                disable-tunnel: w663 -> [_ w694]
                                frame Disabled {
                                n183 = call "envoi mail valves expediées.vi"("tab histo filtré\n par n° cmde"=w691, "DIVISION"=w690, "error in (no error)"=w693, "DATA cmde"=w688, "chaine valves"=w689) -> ("error out"=w692:errorcluster)  [unwired: 6 in]
                                }
                                frame Enabled {
                                n184 = call "Emballage_NumSerie.vi"("Error in"=w696, "Tableau n° valves"=w694) -> ("Error out"=w695:errorcluster)  [unwired: 9 in]
                                }
                                }
                                }
                              }
                              n185 = Build Array (concatenate)(w575, w601) -> (w600:string[])
                            }
                          }
                          "Numéro carton" <- w538
                          n186 = Wait (ms)(milliseconds to wait=1000) -> ()  [unwired: 1 out]
                          n187 = Or(x=w530, y=w500) -> (x .or. y?=w542:bool)
                        }
                        frame True {
                          # "erreur ou recommencer ou visualisation"
                          # "pièces emballées"
                          # "Pas afficher si en mode lecture\nde donnée, sélectionner lorsque\nle mot de passe est demandé."
                          n188 = case shown="True" TRUE {
                            tunnel: w712 -> [w716 w718]
                            tunnel: [w715 w718] -> w710
                            frame False {
                              n189 = call "Emballage_BDD_ON_OFF_Lecteur.vi"("Error in"=w716, "ON/OFF lecteur"=enum_ON_OFF_Lecteur."OFF") -> ("Error out"=w715:errorcluster)  [unwired: 7 in, 2 out]
                            }
                            frame True {
                            }
                          }
                          n190 = call "Afficher un message à l'utilisateur2"("error in (no error)"=w710, "Enable"=FALSE, "Message"="Rien n'a été scanné.\nScanner à nouveau") -> ("error out"=w698:errorcluster)  [unwired: 7 in, 1 out]
                          n191 = Compound Arithmetic op=OR("quitter", w703) -> (w701:bool)
                        }
                      }
                      n192 = case shown="True" "Certificat" {
                        tunnel: w406 -> [_ w450]
                        frame False {
                        }
                        frame True {
                          n193 = call "Emballage_BDD_option_Certificat.vi"("Error in"=w450) -> ("Error out"=w452:errorcluster)  [unwired: 10 in]
                          n194 = property on="Certificat" class="Bool (strict)"(error in=w452, "Value"=FALSE) -> ()  [unwired: 1 in, 2 out]
                        }
                      }
                      n195 = case shown="True" "carton" {
                        tunnel: w406 -> [w472 w476]
                        tunnel: [w472 w474] -> w420
                        tunnel: w403 -> [_ w473]
                        frame False {
                        }
                        frame True {
                          n196 = call "emballage affiche le contenu du carton_FLAT.vi"("Tableau \nlots OUT"=w473, "error in"=w476) -> ("error out"=w475:errorcluster)  [unwired: 4 in]
                          n197 = property on="carton" class="Bool (strict)"(error in=w475, "Valeur"=FALSE) -> (error out=w474:errorcluster)  [unwired: 1 in, 1 out]
                        }
                      }
                      n198 = case shown="True" "EC emballage" {
                        tunnel: w410 -> [_ w479]
                        frame False {
                        }
                        frame True {
                          n199 = call "emballage affiche série en cours.vi"("chaîne 2D"=w479) -> ("error out"=w478:errorcluster)  [unwired: 1 in]
                          n200 = property on="EC emballage" class="Bool (strict)"(error in=w478, "Valeur"=FALSE) -> ()  [unwired: 1 in, 2 out]
                        }
                      }
                      n201 = case shown="True" "Imprimer n° cmde" {
                        tunnel: [w453 w456] -> w416
                        tunnel: w420 -> [w453 w455]
                        tunnel: "00000/00-01.01.01" ("n° commande") -> [_ w454]
                        frame False {
                        }
                        frame True {
                          n202 = call "Imprimer les n° d'une cmde.vi"("error in (no error)"=w455, "n° commande"=w454) -> ("error IO"=w457:errorcluster)  [unwired: 3 in]
                          n203 = property on="Imprimer n° cmde" class="Bool (strict)"(error in=w457, "Valeur"=FALSE) -> (error out=w456:errorcluster)  [unwired: 1 in, 1 out]
                        }
                      }
                      n204 = Unbundle By Name(w416) -> ("status"=w415:bool)
                      n205 = Or(x=w415, y=w417) -> (x .or. y?=w405:bool)
                    }
                  }
                  frame True {
                    w722 = -1
                    # "pièces emballées"
                    n206 = call "03_FS_GFV_Logfile.vi"("Chaîne"="annuler de nvl serie ou pb GPAO", "States"=60_FS_SetGet."set") -> ()  [unwired: 8 in, 2 out]
                  }
                }
                "largeur index" <- w371
                "offset sur code \nbar début index" <- w370
                "pièces EC emballées" <- w373
                "arreterSerie" <- w367
                n207 = local write "Numéro carton"(w365) -> ()
                n208 = local write "Nombre de pièce"(w366) -> ()
              }
              frame "LecteurOFF" {
                n209 = call "Emballage_BDD_GVF_DATACMD.vi"("SetGet"=60_FS_SetGet."get") -> ("Annuler new série (T=OK) OUT"=w729:bool)  [unwired: 7 in, 7 out]
                n210 = case shown="False" w729 {
                  tunnel: [w766 errorcluster {"status"=FALSE, "code"=0, "source"=""} ("error out")] -> w730
                  frame False {
                    n211 = disable-structure shown="Par défaut" {
                      disable-tunnel: [w769 errorcluster {"status"=FALSE, "code"=0, "source"=""} ("error out")] -> w766
                      frame condition #0 (active) {
                        n212 = call "Emballage_BDD_ON_OFF_Lecteur.vi"("Error in"=errorcluster {"status"=FALSE, "code"=0, "source"=""}, "ON/OFF lecteur"=enum_ON_OFF_Lecteur."OFF (open/Close)") -> ("Error out"=w769:errorcluster)  [unwired: 7 in, 2 out]
                      }
                      frame condition #1 {
                      }
                    }
                  }
                  frame True {
                  }
                }
                n213 = disable-structure shown="Désactivé" {
                  disable-tunnel: w730 -> [w743 w765]
                  disable-tunnel: [w733 w765] -> w726
                  frame Disabled {
                    n214 = local read "pièces EC emballées"() -> (w736:string)
                    n215 = local read "recommencer la cmde EC"() -> (w737:bool)
                    n216 = local read "Continuer l'emballage"() -> (w732:bool)
                    n217 = call "Emballage_BDD_GVF_bool_Réseau_annule_visualiser.vi"("SetGet"=60_FS_SetGet."get") -> ("Visualiser OUT"=w735:bool)  [unwired: 12 in, 2 out]
                    n218 = Match Pattern(string=w736, regular expression="/" ("expression régulière")) -> (after substring=w739:string)  [unwired: 1 in, 3 out]
                    n219 = Not Equal?(x=w739, y="" ("result string")) -> (x != y?=w741:bool)
                    n220 = And(x=w735, y=w741) -> (x .and. y?=w742:bool)
                    n221 = Compound Arithmetic op=OR ("Opérateur arithmétique")(w742, w737, w732) -> (w731:bool)
                    n222 = case shown="True" w731 {
                      tunnel: w743 -> [w744 w748]
                      tunnel: [w744 w755] -> w733
                      frame False {
                      }
                      frame True {
                        # "Supprime ligne de cmde non terminée"
                        n223 = call "Emballage_BDD_GVF_chemin_TXT.vi"("Error in"=w748, "Énum"=enum16{"get", "set"}."get") -> ("Error out"=w747:errorcluster, "Produits_Commandes_en_cours.txt OUT"=w746:path)  [unwired: 8 in]
                        n224 = Read from Text File(file (use dialog)=w746, error in=w747) -> (text=w752:string, error out=w750:errorcluster)  [unwired: 2 in, 2 out]
                        n225 = local read "index commande en cours"() -> (w745:i32)
                        n226 = Spreadsheet String To Array(format string="%s", spreadsheet string=w752, array type (2D Dbl)=string[][] []) -> (array=w751:string[][])  [unwired: 1 in]
                        n227 = Open/Create/Replace File(file path (use dialog)=w746, error in=w750, operation (0:open)=T6."replace" ("opération (0 : open)")) -> (refnum out=w761:refnum<file>, error out=w757:errorcluster)  [unwired: 3 in, 1 out]
                        n228 = Delete From Array(array=w751, length=1 ("longueur"), index (row)=w745) -> (array with subset deleted=w759:string[][])  [unwired: 1 in, 1 out]
                        n229 = Array To Spreadsheet String(array=w759, 3:"%s") -> (spreadsheet string=w758:string)  [unwired: 1 in]
                        n230 = Write to Text File(file (use dialog)=w761, text=w758, error in=w757) -> (refnum out=w762:refnum<file>, error out=w756:errorcluster)  [unwired: 1 in, 1 out]
                        n231 = Close File(refnum=w762, error in=w756) -> (error out=w755:errorcluster)  [unwired: 1 out]
                      }
                    }
                  }
                  frame Enabled {
                    # "#LTI 20180905:\nplus utilisation cmd en cours.txt"
                  }
                }
              }
              frame "SaveData" {
                # "Sauvegarde des données"
                n232 = call "Emballage_BDD_GVF_bool_Réseau_annule_visualiser.vi"("SetGet"=60_FS_SetGet."get") -> ("Visualiser OUT"=w776:bool)  [unwired: 12 in, 2 out]
                n233 = case shown="False" w776 {
                  tunnel: [w784 FALSE] -> w772
                  tunnel: [w783 w851] -> w777
                  frame False {
                    n234 = local read "arreterSerie"() -> (w782:bool)
                    n235 = call "Emballage_BDD_GVF_DATACMD.vi"("SetGet"=60_FS_SetGet."get") -> ("Annuler new série (T=OK) OUT"=w781:bool)  [unwired: 7 in, 7 out]
                    n236 = Or(x=w781, y=w782) -> (x .or. y?=w779:bool)
                    n237 = case shown="False" w779 {
                      tunnel: [FALSE w801] -> w784
                      tunnel: [w786 w803] -> w783
                      frame False {
                        # "Série fini normalement"
                        n238 = local read "recommencer la cmde EC"() -> (w785:bool)
                        n239 = case shown="True" w785 {
                          tunnel: [errorcluster {"status"=FALSE, "code"=0, "source"=""} ("error out 2") w800] -> w786
                          frame False {
                          }
                          frame True {
                            # "valves supprimées sous la CMDE à recommencer"
                            n240 = call "Emballage_BDD_GVF_DATACMD.vi"("SetGet"=60_FS_SetGet."get", "Error in"=errorcluster {"status"=FALSE, "code"=0, "source"=""}) -> ("No commande FAS OUT"=w790:string, "Error out"=w797:errorcluster)  [unwired: 6 in, 6 out]
                            n241 = Match Pattern(string=w790, regular expression="R" ("expression régulière")) -> (after substring=w792:string, offset past match=w793:i32)  [unwired: 1 in, 2 out]
                            n242 = Equal?(x=w793, y=-1) -> (x = y?=w791:bool)
                            n243 = Select(t=w790, s=w791, f=w792) -> (s? t:f=w789:string)
                            n244 = call "Emballage_BDD_Suppression_SQL_Cmd.vi"("error in (no error)"=w797, "NO_CDEVAL"=w789, "Table (PRODUIT_EMBALLAGE)"="PRODUIT_EMBALLAGE" ("Table")) -> ("error out"=w800:errorcluster)  [unwired: 8 in]
                          }
                        }
                      }
                      frame True {
                        # "pas de sauvegarde si annulation de nvl serie mais sauve commande en cours si pas finie"
                        n245 = local read "Commande interne"() -> (w802:bool)
                        n246 = case shown="False" w802 {
                          tunnel: [w805 w840] -> w803
                          tunnel: [FALSE FALSE] -> w801
                          frame False {
                            # "contrôle si cmd en cours"
                            n247 = disable-structure shown="Enabled" {
                              disable-tunnel: [w810 errorcluster {"status"=FALSE, "code"=0, "source"=""} ("error out")] -> w805
                              frame Disabled {
                                n248 = local read "Nombre de pièce"() -> (w806:i16)
                                n249 = local read "pièces EC emballées"() -> (w807:string)
                                n250 = call "Emballage_BDD_GVF_DATACMD.vi"("SetGet"=60_FS_SetGet."get") -> ("Quantité de la commande OUT"=w809:i32)  [unwired: 7 in, 7 out]
                                n251 = Match Pattern(string=w807, regular expression="/" ("expression régulière")) -> (after substring=w811:string)  [unwired: 1 in, 3 out]
                                n252 = Not Equal?(x=w811, y="" ("result string")) -> (x != y?=w815:bool)
                                n253 = Less?(x=w806, y=w809) -> (x < y?=w814:bool)
                                n254 = And(x=w815, y=w814) -> (x .and. y?=w813:bool)
                                n255 = case shown="True" w813 {
                                tunnel: w807 -> [_ w832]
                                tunnel: w806 -> [_ w830]
                                tunnel: [errorcluster {"status"=FALSE, "code"=0, "source"=""} ("error out") w821] -> w810
                                frame False {
                                }
                                frame True {
                                w833 = string[][] []  # Cst tab
                                n256 = call "Emballage_BDD_GVF_chemin_TXT.vi"("Énum"=enum16{"get", "set"}."get") -> ("Error out"=w818:errorcluster, "Produits_Commandes_en_cours.txt OUT"=w820:path)  [unwired: 9 in]
                                n257 = Open/Create/Replace File(file path (use dialog)=w820, error in=w818, operation (0:open)=T6."open" ("opération (0 : open)")) -> (refnum out=w827:refnum<file>, error out=w823:errorcluster)  [unwired: 3 in, 1 out]
                                n258 = Spreadsheet String To Array(format string="%s", spreadsheet string=w832, array type (2D Dbl)=w833) -> (array=w831:string[][])  [unwired: 1 in]
                                n259 = Set File Position(refnum=w827, from (0:start)=enum16{"start", "end", "current"}."end" ("à partir de (0 : start)"), error in=w823) -> (refnum out=w826:refnum<file>, error out=w822:errorcluster)  [unwired: 1 in]
                                n260 = call "emballage mise en forme pour commandes en cours.vi"("Nb pièces emballées"=w830, "pièces emballées"=w831) -> ("Chaîne pour fichier cmde"=w829:string)  [unwired: 1 in]
                                n261 = Write to Text File(file (use dialog)=w826, text=w829, error in=w822) -> (refnum out=w824:refnum<file>)  [unwired: 1 in, 2 out]
                                n262 = Close File(refnum=w824) -> (error out=w821:errorcluster)  [unwired: 1 in, 1 out]
                                }
                                }
                              }
                              frame Enabled {
                                # "#LTI 20210602\nstop à Faux car après une commande,\nle programme ira dans Choix de référence suivant\npour éviter le chargement des données entre chaque commande"
                                # "#LTI 20180905:\nplus utilisation cmd en cours.txt"
                              }
                            }
                          }
                          frame True {
                            # "cmd interne"
                            n263 = while {
                              shift-right: [w849] -> w842
                              shift-left: errorcluster {"status"=FALSE, "code"=0, "source"=""} ("Error in") -> [w850]
                              stop <- w848 continue-if-true
                              n264 = call "EMBALLAGE_BDD_FichiersSQLEnregistres.vi"("Error in"=w850) -> ("Error out"=w849:errorcluster, "Dans la gamme ?"=w848:bool)  [unwired: 9 in]
                              n265 = Wait (ms)(milliseconds to wait=u32 100 ("attente (ms)")) -> ()  [unwired: 1 out]
                            }
                            n266 = call "Emballage_BDD_GVF_DATACMD.vi"("SetGet"=60_FS_SetGet."get", "Error in"=w842) -> ("DATA cmde OUT"=w846:T3, "Error out"=w845:errorcluster)  [unwired: 6 in, 6 out]
                            n267 = Unbundle By Name(w846) -> ("n° cmde FAS"=w839:string)
                            n268 = call "Emballage_BDD_lectureSQL_Liste PièceDansCmd.vi"("Error in"=w845, "NO_CDEVAL"=w839) -> ("Error out"=w841:errorcluster, "Liste n° pièces de la cmde"=w844:string[])  [unwired: 5 in, 3 out]
                            n269 = Array Size(array=w844) -> (size(s)=w838:i32)
                            n270 = call "Emballage_BDD_afficheInfoCmdInterne.vi"("Error in"=w841, "nbr de pièce"=w838, "CMD interne"=w839) -> ("Error out"=w840:errorcluster)  [unwired: 8 in]
                          }
                        }
                      }
                    }
                  }
                  frame True {
                    # "rend visible affichage scanner"
                    # "pas sauvegarde si en mode visualisation"
                    n271 = property on="Numéro scanné" class="Str"(error in=errorcluster {"status"=FALSE, "code"=0, "source"=""} ("error out"), "Visible"=TRUE) -> (error out=w851:errorcluster)  [unwired: 1 in, 1 out]
                  }
                }
                n272 = property on="quitter" class="Bool (strict)"(error in=w777, "Valeur"=FALSE) -> (error out=w774:errorcluster)  [unwired: 1 in, 1 out]
              }
              frame "ChoixProduit" {
                n273 = call "Emballage_BDD_choix_Config.vi"("Error in"=w858) -> ("Error out"=w860:errorcluster, "Arrêt programme?"=w855:bool)  [unwired: 7 in, 2 out]
                n274 = property on="Numéro scanné" class="Str"(error in=w860, "Visible"=TRUE) -> (error out=w857:errorcluster)  [unwired: 1 in, 1 out]
              }
            }
            n275 = Unbundle By Name(w35) -> ("status"=w34:bool)
            n276 = Or(x=w34, y=w32) -> (x .or. y?=w33:bool)
            "Etat" <- w28
            "NumSem" <- 0.0 ("NumSem")
          }
        }
        frame Error {
          n277 = call "03_FS_GFV_Logfile.vi"("Chaîne"="erreur après initialisation des variables", "States"=60_FS_SetGet."set") -> ()  [unwired: 8 in, 2 out]
        }
      }
    }
    frame Error {
      n278 = call "03_FS_GFV_Logfile.vi"("Chaîne"="erreur après \"rétablirValParDefaut\"", "States"=60_FS_SetGet."set") -> ()  [unwired: 8 in, 2 out]
    }
  }
  "error out" <- w5
  n279 = case shown="Error" w5 {
    selector: w5 -> [_ w873]
    tunnel: [TRUE TRUE] -> w11
    frame No Error {
    }
    frame Error {
      n280 = Unbundle By Name(w873) -> ("source"=w868:string)
      n281 = Concatenate Strings("Erreur emballage: " ("chaîne"), w868) -> (w871:string)
      n282 = call "03_FS_GFV_Logfile.vi"("Chaîne"=w871, "States"=60_FS_SetGet."set") -> ()  [unwired: 8 in, 2 out]
    }
  }
  n283 = call "Emballage_BDD_GVF_softSAFE.vi"("Énum"=enum16{"SET", "GET"}."SET", "SOFTSAFE"=w11) -> ()  [unwired: 1 in, 2 out]
